vi "MS time axis from date-time values.vi"(0 "Reference":string, 1 "Time":string) -> (2 "Ref time stamp":timestamp, 3 "dt /s":dbl, 4 "Time stamp":timestamp)   [LabVIEW 2015]
uses:
  <vilib>/Utility/miscctls.llb/LVDateTimeRec.ctl
panel:
  in  "date time rec":T1
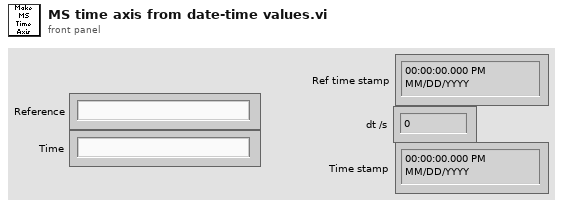
[diagram p1: front panel]
types:
  T1 = typedef "LVDateTimeRec.ctl" = cluster{"fractional second":dbl, "second":i32, "minute":i32, "hour":i32, "day of month":i32, "month":i32, "year":i32, "day of week":i32, "day of year":i32, "DST":i32}
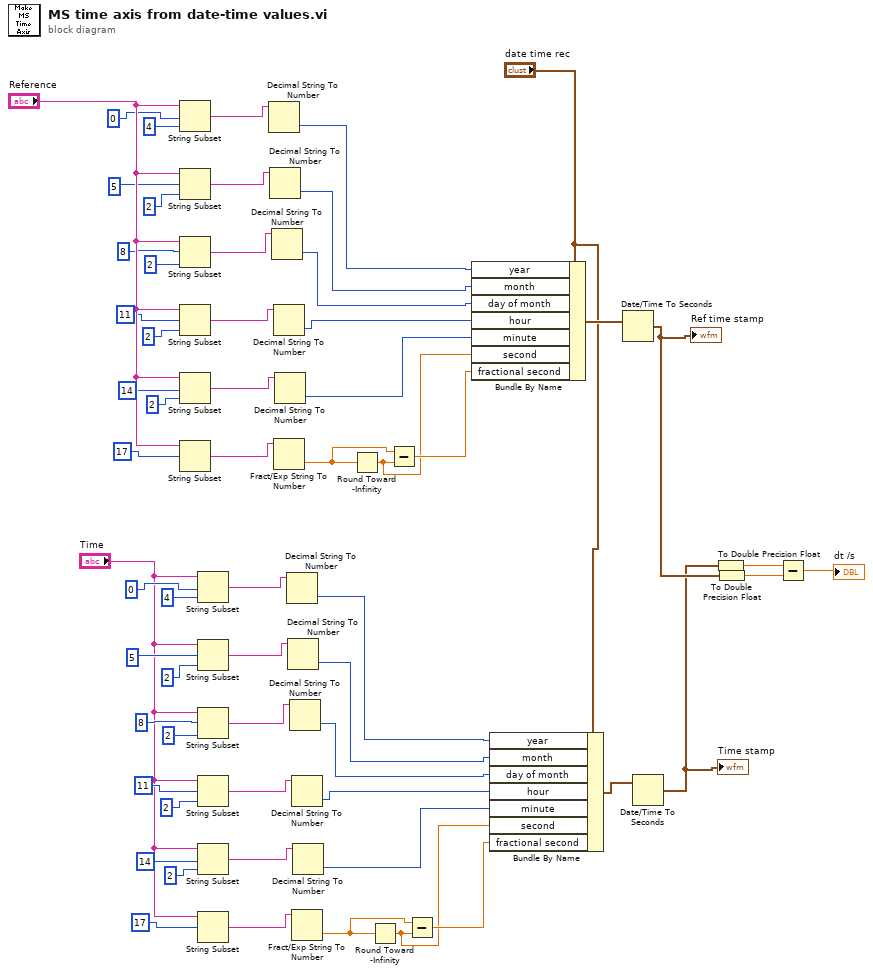
[diagram p0: block diagram]
diagram:
  n1 = String Subset(string="Reference", offset (0)=0, length (rest)=4) -> (substring=w48:string)
  n2 = String Subset(string="Reference", offset (0)=5, length (rest)=2) -> (substring=w47:string)
  n3 = String Subset(string="Reference", offset (0)=8, length (rest)=2) -> (substring=w46:string)
  n4 = String Subset(string="Reference", offset (0)=11, length (rest)=2) -> (substring=w45:string)
  n5 = String Subset(string="Reference", offset (0)=14, length (rest)=2) -> (substring=w44:string)
  n6 = String Subset(string="Reference", offset (0)=17) -> (substring=w43:string)  [unwired: 1 in]
  n7 = String Subset(string="Time", offset (0)=0, length (rest)=4) -> (substring=w22:string)
  n8 = String Subset(string="Time", offset (0)=5, length (rest)=2) -> (substring=w21:string)
  n9 = String Subset(string="Time", offset (0)=8, length (rest)=2) -> (substring=w20:string)
  n10 = String Subset(string="Time", offset (0)=11, length (rest)=2) -> (substring=w19:string)
  n11 = String Subset(string="Time", offset (0)=14, length (rest)=2) -> (substring=w18:string)
  n12 = String Subset(string="Time", offset (0)=17) -> (substring=w17:string)  [unwired: 1 in]
  n13 = Decimal String To Number(string=w48) -> (number=w35:i32)  [unwired: 2 in, 1 out]
  n14 = Decimal String To Number(string=w47) -> (number=w36:i32)  [unwired: 2 in, 1 out]
  n15 = Decimal String To Number(string=w46) -> (number=w37:i32)  [unwired: 2 in, 1 out]
  n16 = Decimal String To Number(string=w45) -> (number=w38:i32)  [unwired: 2 in, 1 out]
  n17 = Fract/Exp String To Number(string=w43) -> (number=w42:dbl)  [unwired: 3 in, 1 out]
  n18 = Decimal String To Number(string=w44) -> (number=w39:i32)  [unwired: 2 in, 1 out]
  n19 = Decimal String To Number(string=w22) -> (number=w9:i32)  [unwired: 2 in, 1 out]
  n20 = Decimal String To Number(string=w21) -> (number=w10:i32)  [unwired: 2 in, 1 out]
  n21 = Decimal String To Number(string=w20) -> (number=w11:i32)  [unwired: 2 in, 1 out]
  n22 = Decimal String To Number(string=w19) -> (number=w12:i32)  [unwired: 2 in, 1 out]
  n23 = Fract/Exp String To Number(string=w17) -> (number=w16:dbl)  [unwired: 3 in, 1 out]
  n24 = Decimal String To Number(string=w18) -> (number=w13:i32)  [unwired: 2 in, 1 out]
  n25 = Round Toward -Infinity(1:w42) -> (0:w40:dbl)
  n26 = Round Toward -Infinity(1:w16) -> (0:w14:dbl)
  n27 = Subtract(x=w42, y=w40) -> (x-y=w41:dbl)
  n28 = Subtract(x=w16, y=w14) -> (x-y=w15:dbl)
  n29 = Bundle By Name(cluster="date time rec", "year"=w35, "month"=w36, "day of month"=w37, "hour"=w38, "minute"=w39, "second"=w40, "fractional second"=w41) -> (w34:T1)
  n30 = Bundle By Name(cluster="date time rec", "year"=w9, "month"=w10, "day of month"=w11, "hour"=w12, "minute"=w13, "second"=w14, "fractional second"=w15) -> (w6:T1)
  n31 = Date/Time To Seconds(2:w34) -> (0:w5:timestamp)  [unwired: 1 in]
  "Ref time stamp" <- w5
  n32 = Date/Time To Seconds(2:w6) -> (0:w4:timestamp)  [unwired: 1 in]
  "Time stamp" <- w4
  n33 = To Double Precision Float(number=w4) -> (double precision float=w2:dbl)
  n34 = To Double Precision Float(number=w5) -> (double precision float=w1:dbl)
  n35 = Subtract(x=w2, y=w1) -> (x-y=→"dt /s":dbl)
